vi "test_Tx Exec Unit (UDP).vi"() -> ()   [LabVIEW 2020]
uses:
  <instrlib>/AIM GmbH/_AIM 664/_controls/comm_config_vl_tx.ctl
  <instrlib>/AIM GmbH/_AIM 664/_controls/comm_udp_tx.ctl
  Shared/Encoding (Arinc664).ctl
  Import/_typedefs/board_setup.ctl
  <vilib>/NI VeriStand/Custom Device API/Custom Device Item Ref.ctl
  Engine/Implementation/Shared Resources/Shared Resources.lvclass
  C:/git/niveristand-aim-arinc664-custom-device/Source/Custom Device Support/Engine/Interfaces/Shared Resources/Shared Resources.lvclass
  Engine/Implementation/Tx UDP Execution Unit/Tx UDP Execution Unit.lvclass
  <vilib>/NI VeriStand/Custom Device API/Custom Device API.lvlib
  <instrlib>/AIM GmbH/_AIM 664/AIM664LV.lvlib
  Import/AIM ARINC 664 Import.lvlib
panel:
  in  "Tab Control":enum32{"Manual", "From File"}(tab)
  in  "tx_udp_vl":T3(array[cluster])=[{"VL Config"={"VlId"=60, "NumOfSubVl"=1, "rate ms [Bag]"=2, "domainID"=2, "sideID"=1, "locationID"=1, "interfaceID"=1, "NetSelect"=3, "Skew"=0, "MaxFrameLength"=559, "FrameBufferSize"=0}, "CommPort Config"=[{"PortType"=enum."FDX_UDP_SAMPLING", "partitionID"=1, "SubVlId"=1, "UdpSrcPort"=24, "UdpDstPort"=23, "SampleRateMs"=2.0, "UdpNumBufMessages"=0, "UdpMaxMessageSize"=512}, {"PortType"=enum."FDX_UDP_SAMPLING", "partitionID"=1, "SubVlId"=1, "UdpSrcPort"=34, "UdpDstPort"=33, "SampleRateMs"=2.0, "UdpNumBufMessages"=0, "UdpMaxMessageSize"=512}]}] {"VL Config"."NetSelect" items=["FDX_TX_FRAME_DLY_A"=0, "FDX_TX_FRAME_DLY_B"=1, "FDX_TX_FRAME_BOTH "=3, "FDX_TX_FRAME_ONLY_A"=4, "FDX_TX_FRAME_ONLY_B "=5]; "VL Config"."interfaceID" format="%.0b"}
  in  "tx_param":T5(array[cluster])=[{"Data"=[0, 0, 0, 0, 0, 0, 0, 0, 0, 0, 0, 0, 0, 0, 0, 0, 0, 0, 0, 0, 0, 0, 0, 0, 0, 0, 0, 0, 0, 0, 0, 0, 0, 0, 0, 0, 0, 0, 0, 0, 0, 0, 0, 0, 0, 0, 0, 0, 0, 0, 0, 0, 0, 0, 0, 0, 0, 0, 0, 0, 0, 0, 0, 0, 0, 0, 0, 0, 0, 0, 0, 0, 0, 0, 0, 0, 0, 0, 0, 0, 0, 0, 0, 0, 0, 0, 0, 0, 0, 0, 0, 0, 0, 0, 0, 0, 0, 0, 0, 0, 0, 0, 0, 0, 0, 0, 0, 0, 0, 0, 0, 0, 0, 0, 0, 0, 0, 0, 0, 0, 0, 0, 0, 0, 0, 0, 0, 0, 0, 0, 0, 0, 0, 0, 0, 0, 0, 0, 0, 0, 0, 0, 0, 0, 0, 0, 0, 0, 0, 0, 0, 0, 0, 0, 0, 0, 0, 0, 0, 0, 0, 0, 0, 0, 0, 0, 0, 0, 0, 0, 0, 0, 0, 0, 0, 0, 0, 0, 0, 0, 0, 0, 0, 0, 0, 0, 0, 0, 0, 0, 0, 0, 0, 0, 0, 0, 0, 0, 0, 0, 0, 0, 0, 0, 0, 0, 0, 0, 0, 0, 0, 0, 0, 0, 0, 0, 0, 0, 0, 0, 0, 0, 0, 0, 0, 0, 0, 0, 0, 0, 0, 0, 0, 0, 0, 0, 0, 0, 0, 0, 0, 0, 0, 0, 0, 0, 0, 0, 0, 0, 0, 0, 0, 0, 0, 0, 0, 0, 0, 0, 0, 0, 0, 0, 0, 0, 0, 0, 0, 0, 0, 0, 0, 0, 0, 0, 0, 0, 0, 0, 0, 0, 0, 0, 0, 0, 0, 0, 0, 0, 0, 0, 0, 0, 0, 0, 0, 0, 0, 0, 0, 0, 0, 0, 0, 0, 0, 0, 0, 0, 0, 0, 0, 0, 0, 0, 0, 0, 0, 0, 0, 0, 0, 0, 0, 0, 0, 0, 0, 0, 0, 0, 0, 0, 0, 0, 0, 0, 0, 0, 0, 0, 0, 0, 0, 0, 0, 0, 0, 0, 0, 0, 0, 0, 0, 0, 0, 0, 0, 0, 0, 0, 0, 0, 0, 0, 0, 0, 0, 0, 0, 0, 0, 0, 0, 0, 0, 0, 0, 0, 0, 0, 0, 0, 0, 0, 0, 0, 0, 0, 0, 0, 0, 0, 0, 0, 0, 0, 0, 0, 0, 0, 0, 0, 0, 0, 0, 0, 0, 0, 0, 0, 0, 0, 0, 0, 0, 0, 0, 0, 0, 0, 0, 0, 0, 0, 0, 0, 0, 0, 0, 0, 0, 0, 0, 0, 0, 0, 0, 0, 0, 0, 0, 0, 0, 0, 0, 0, 0, 0, 0, 0, 0, 0, 0, 0, 0, 0, 0, 0, 0, 0, 0, 0, 0, 0, 0, 0, 0, 0, 0, 0, 0, 0, 0, 0, 0, 0, 0, 0, 0, 0, 0, 0, 0, 0, 0, 0, 0, 0, 0, 0, 0, 0, 0, 0, 0, 0, 0, 0, 0, 0, 0, 0, 0, 0, 0, 0, 0, 0, 0, 0], "Parameters"=[{"start index"=0, "size"=64, "encoding"=6, "signed"=TRUE, "scale multiplier"=1.0, "scale offset"=0.0}, {"start index"=64, "size"=64, "encoding"=6, "signed"=TRUE, "scale multiplier"=1.0, "scale offset"=0.0}]}, {"Data"=[0, 0, 0, 0, 0, 0, 0, 0, 0, 0, 0, 0, 0, 0, 0, 0, 0, 0, 0, 0, 0, 0, 0, 0, 0, 0, 0, 0, 0, 0, 0, 0, 0, 0, 0, 0, 0, 0, 0, 0, 0, 0, 0, 0, 0, 0, 0, 0, 0, 0, 0, 0, 0, 0, 0, 0, 0, 0, 0, 0, 0, 0, 0, 0, 0, 0, 0, 0, 0, 0, 0, 0, 0, 0, 0, 0, 0, 0, 0, 0, 0, 0, 0, 0, 0, 0, 0, 0, 0, 0, 0, 0, 0, 0, 0, 0, 0, 0, 0, 0, 0, 0, 0, 0, 0, 0, 0, 0, 0, 0, 0, 0, 0, 0, 0, 0, 0, 0, 0, 0, 0, 0, 0, 0, 0, 0, 0, 0, 0, 0, 0, 0, 0, 0, 0, 0, 0, 0, 0, 0, 0, 0, 0, 0, 0, 0, 0, 0, 0, 0, 0, 0, 0, 0, 0, 0, 0, 0, 0, 0, 0, 0, 0, 0, 0, 0, 0, 0, 0, 0, 0, 0, 0, 0, 0, 0, 0, 0, 0, 0, 0, 0, 0, 0, 0, 0, 0, 0, 0, 0, 0, 0, 0, 0, 0, 0, 0, 0, 0, 0, 0, 0, 0, 0, 0, 0, 0, 0, 0, 0, 0, 0, 0, 0, 0, 0, 0, 0, 0, 0, 0, 0, 0, 0, 0, 0, 0, 0, 0, 0, 0, 0, 0, 0, 0, 0, 0, 0, 0, 0, 0, 0, 0, 0, 0, 0, 0, 0, 0, 0, 0, 0, 0, 0, 0, 0, 0, 0, 0, 0, 0, 0, 0, 0, 0, 0, 0, 0, 0, 0, 0, 0, 0, 0, 0, 0, 0, 0, 0, 0, 0, 0, 0, 0, 0, 0, 0, 0, 0, 0, 0, 0, 0, 0, 0, 0, 0, 0, 0, 0, 0, 0, 0, 0, 0, 0, 0, 0, 0, 0, 0, 0, 0, 0, 0, 0, 0, 0, 0, 0, 0, 0, 0, 0, 0, 0, 0, 0, 0, 0, 0, 0, 0, 0, 0, 0, 0, 0, 0, 0, 0, 0, 0, 0, 0, 0, 0, 0, 0, 0, 0, 0, 0, 0, 0, 0, 0, 0, 0, 0, 0, 0, 0, 0, 0, 0, 0, 0, 0, 0, 0, 0, 0, 0, 0, 0, 0, 0, 0, 0, 0, 0, 0, 0, 0, 0, 0, 0, 0, 0, 0, 0, 0, 0, 0, 0, 0, 0, 0, 0, 0, 0, 0, 0, 0, 0, 0, 0, 0, 0, 0, 0, 0, 0, 0, 0, 0, 0, 0, 0, 0, 0, 0, 0, 0, 0, 0, 0, 0, 0, 0, 0, 0, 0, 0, 0, 0, 0, 0, 0, 0, 0, 0, 0, 0, 0, 0, 0, 0, 0, 0, 0, 0, 0, 0, 0, 0, 0, 0, 0, 0, 0, 0, 0, 0, 0, 0, 0, 0, 0, 0, 0, 0, 0, 0, 0, 0, 0, 0, 0, 0, 0, 0, 0, 0, 0, 0, 0, 0, 0, 0, 0, 0, 0, 0, 0, 0, 0, 0, 0, 0, 0, 0, 0, 0, 0, 0, 0, 0, 0, 0, 0], "Parameters"=[{"start index"=0, "size"=64, "encoding"=6, "signed"=TRUE, "scale multiplier"=1.0, "scale offset"=0.0}, {"start index"=64, "size"=64, "encoding"=6, "signed"=TRUE, "scale multiplier"=1.0, "scale offset"=0.0}]}] {"Parameters"."encoding" items=["BNR", "BCD", "Discrete"]}
  in  "Tx_UDP_Frames file path":path=path "/home/admin/Port_0_Tx_UDP_Frames.bin"
  out "Frame parse error":errorcluster caption="error out"
  in  "Tx_UDP_VLs file path":path=path "/home/admin/Port_0_Tx_UDP_VLs.bin"
  in  "Update data every N calls":i32=1
  out "# of outs":i32=1
  in  "# of ins":i32=1
  out "exec time us":cluster{u32, u32}(graph)={659, 311}
  in  "Init Shared Resources":bool=TRUE
  in  "shared resources":T6 {"portConfig" items=["FDX_SINGLE", "FDX_REDUNDANT"]; "portSpeed" items=["FDX_100MBIT", "FDX_10MBIT", "FDX_AUTO_100MBIT", "FDX_AUTO_10MBIT", "FDX_AUTO_ERROR", "FDX_1000MBIT"]}
  in  "new element/subarray":dbl[](array[numeric])
  in  "port id":u32
  in  "board id":u32
  in  "loop rate mS":u32=10
  in  "stop":bool
  out "Values out":dbl[](array[numeric])=[1.0]
  out "error out":errorcluster
  # "Once running, switch to Manual tabl to see what has been uploaded from file"
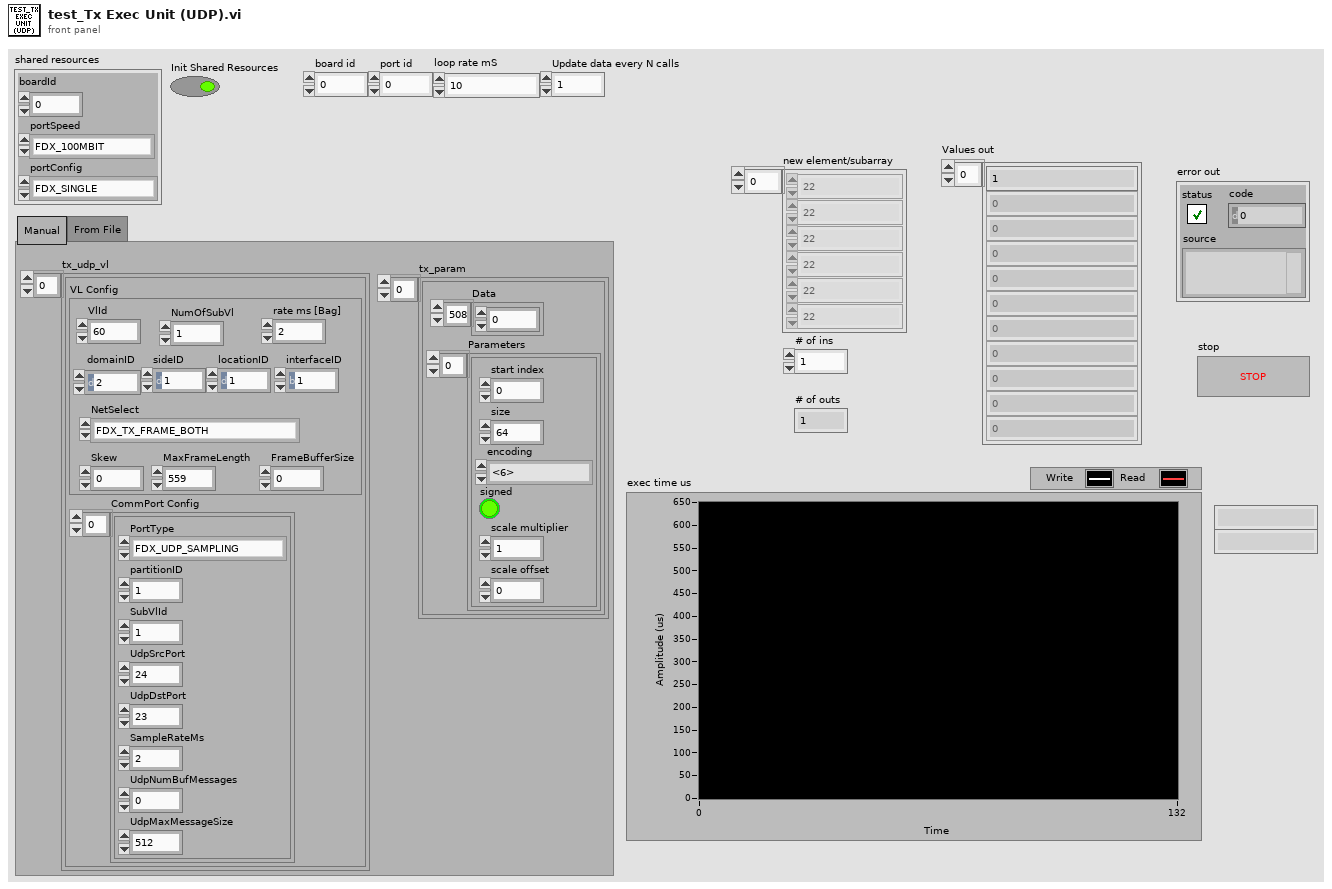
[diagram p1: front panel]
types:
  T1 = typedef "AIM664LV.lvlib/comm_config_vl_tx.ctl" = cluster{"VlId":u16, "NumOfSubVl":u16, "rate ms [Bag]":u32, "domainID":u8, "sideID":u8, "locationID":u8, "interfaceID":u8, "NetSelect":u32, "Skew":u32, "MaxFrameLength":u32, "FrameBufferSize":u32}
  T2 = typedef "AIM664LV.lvlib/comm_udp_tx.ctl" = cluster{"PortType":enum16{"FDX_UDP_SAMPLING", "FDX_UDP_QUEUING"}, "partitionID":u8, "SubVlId":u8, "UdpSrcPort":u16, "UdpDstPort":u16, "SampleRateMs":dbl, "UdpNumBufMessages":u32, "UdpMaxMessageSize":u32}
  T3 = cluster{"VL Config":T1, "CommPort Config":T2[]}[]
  T4 = typedef "Encoding (Arinc664).ctl" = u16
  T5 = cluster{"Data":u8[], "Parameters":cluster{"start index":i32, "size":i32, "encoding":T4, "signed":bool, "scale multiplier":dbl, "scale offset":dbl}[]}[]
  T6 = typedef "AIM ARINC 664 Import.lvlib/board_setup.ctl" = cluster{"boardId":u32, "portSpeed":u32, "portConfig":u32}
  T7 = typedef "Custom Device API.lvlib/Custom Device Item Ref.ctl" = u64
  T8 = cluster{"start index":i32, "size":i32, "encoding":T4, "signed":bool, "scale multiplier":dbl, "scale offset":dbl}[]
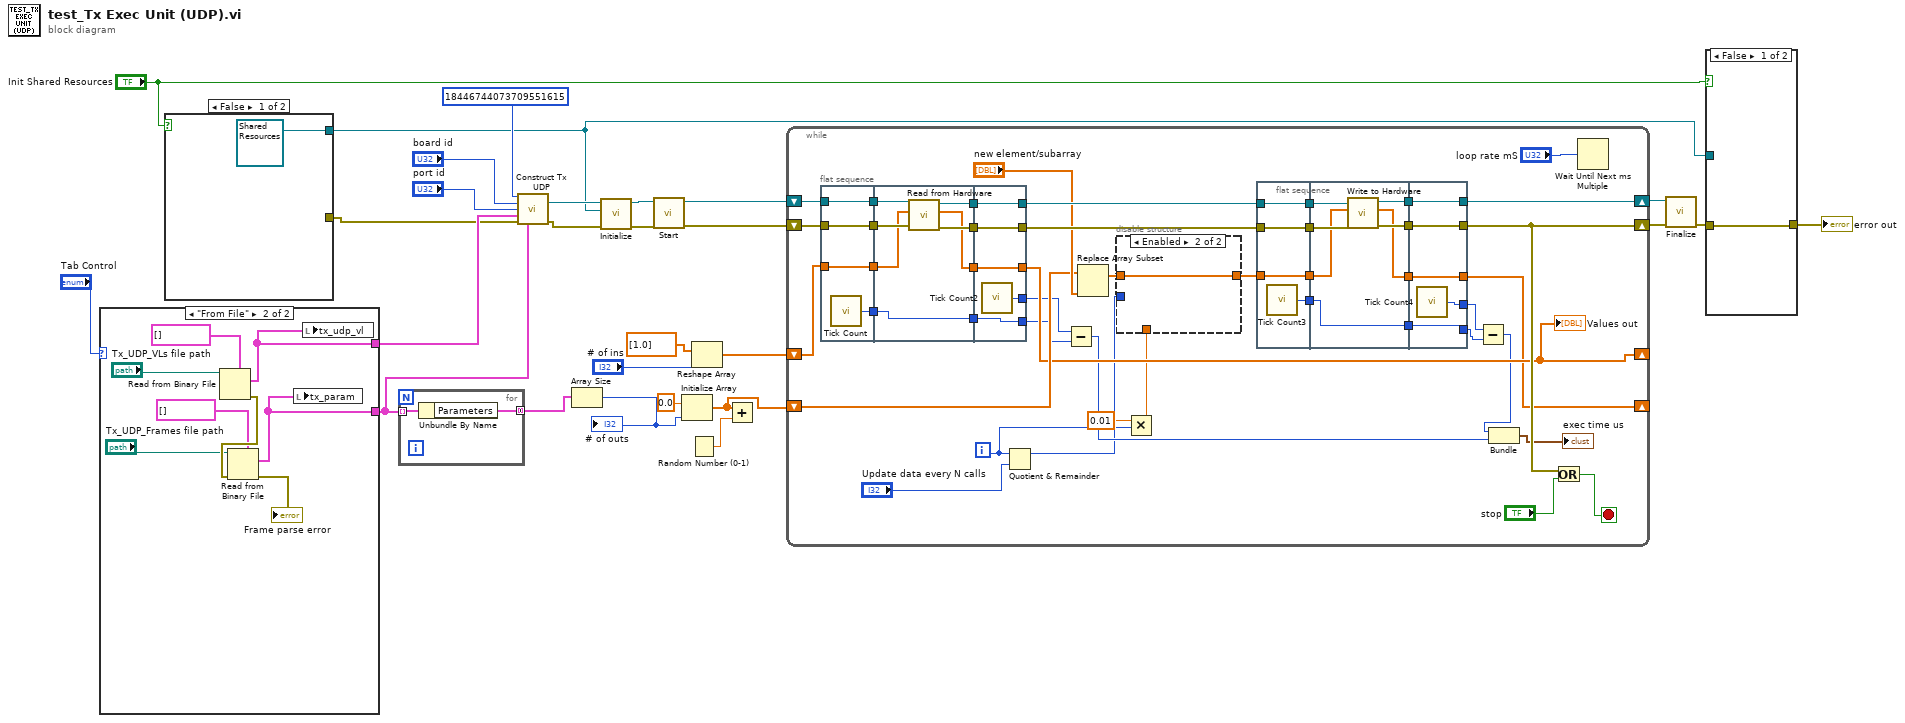
[diagram p0: block diagram]
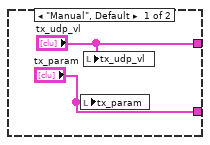
[diagram p2: hidden frame]
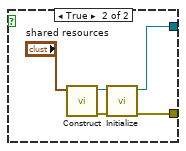
[diagram p3: hidden frame]
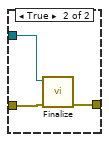
[diagram p4: hidden frame]
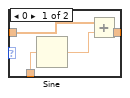
[diagram p6: hidden frame]
diagram:
  n1 = case shown="\"From File\"" "Tab Control" {
    tunnel: ["tx_udp_vl" w31] -> w18
    tunnel: ["tx_param" w30] -> w2
    frame "Manual", Default {
      n2 = local write "tx_param"("tx_param") -> ()
      n3 = local write "tx_udp_vl"("tx_udp_vl") -> ()
    }
    frame "From File" {
      n4 = Read from Binary File(5:T3 [] ("tx_udp_vl"), 11:"Tx_UDP_VLs file path") -> (0:w36:errorcluster, 2:w31:T3)  [unwired: 4 in, 2 out]
      n5 = Read from Binary File(5:T5 [] ("tx_param"), 8:w36, 11:"Tx_UDP_Frames file path") -> (0:→"Frame parse error":errorcluster, 2:w30:T5)  [unwired: 3 in, 2 out]
      n6 = local write "tx_param"(w30) -> ()
      n7 = local write "tx_udp_vl"(w31) -> ()
    }
  }
  n8 = case shown="False" "Init Shared Resources" {
    tunnel: [refnum<class "Shared Resources.lvclass"> refnum ("Shared Resources out") w41] -> w11
    tunnel: [_ w40] -> w15
    frame False {
    }
    frame True {
      n9 = call "Construct.vi"("board properties in"="shared resources") -> ("error out"=w42:errorcluster, "Shared Resources out"=w43:refnum<class "Shared Resources.lvclass">)  [unwired: 9 in]
      n10 = call-dynamic "Initialize.vi"("error in"=w42, "Shared Resources in"=w43) -> ("error out"=w40:errorcluster, "Shared Resources out"=w41:refnum<class "Shared Resources.lvclass">)  [unwired: 8 in]
    }
  }
  n11 = for {
    tunnel: [w45] -> w8 mode=concatenating
    tunnel: w2 -> [w44] mode=indexing
    n12 = Unbundle By Name(w44) -> ("Parameters"=w45:T8)
  }
  n13 = call "Construct Tx UDP.vi"("custom device ref in"=T7 18446744073709551615, "InstrumentHandle_board"="board id", "InstrumentHandle_port"="port id", "VL Configurations"=w18, "error in (no error)"=w15, "CommPort Payload"=w2) -> ("Execution Unit Out"=w21:refnum<class "Tx UDP Execution Unit.lvclass">, "error out"=w20:errorcluster)  [unwired: 7 in, 1 out]
  n14 = Array Size(array=w8) -> (size(s)=w7:i32)
  "# of outs" <- w7
  n15 = call-dynamic "Initialize.vi"("error in"=w20, "shared resources"=w11, "Tx UDP Execution Unit in"=w21) -> ("error out"=w27:errorcluster, "Tx UDP Execution Unit out"=w22:refnum<class "Tx UDP Execution Unit.lvclass">)  [unwired: 7 in]
  n16 = call-dynamic "Start.vi"("error in"=w27, "Tx UDP Execution Unit in"=w22) -> ("error out"=w24:errorcluster, "Tx UDP Execution Unit out"=w23:refnum<class "Tx UDP Execution Unit.lvclass">)  [unwired: 8 in]
  n17 = Initialize Array(0.0 ("Value"), w7) -> (w4:dbl[])
  n18 = Random Number (0-1)() -> (number: 0 to 1=w5:dbl)
  n19 = Reshape Array(dbl[] [1.0] ("Values in"), "# of ins") -> (w9:dbl[])
  n20 = Add(x=w4, y=w5) -> ()  [unwired: 1 out]
  n21 = while {
    shift-right: [w85] -> w25
    shift-left: w23 -> [w89]
    shift-right: [w83] -> w26
    shift-left: w24 -> [w88]
    shift-right: [w70] -> _
    shift-left: w9 -> [w73]
    shift-right: [w63] -> _
    shift-left: w4 -> [w74]
    i -> [w48]
    stop <- w81 stop-if-true
    n22 = flat-sequence {
      tunnel: w88 -> [w102]
      tunnel: w89 -> [w103]
      tunnel: [w103] -> w78
      tunnel: [w102] -> w77
      tunnel: w73 -> [w101]
      tunnel: [w101] -> w72
      tunnel: [w100] -> w59
      tunnel: w78 -> [w110]
      tunnel: w77 -> [w109]
      tunnel: [w108] -> w76
      tunnel: [w107] -> w75
      tunnel: w72 -> [w106]
      tunnel: [w105] -> w71
      tunnel: [w104] -> w60
      tunnel: w59 -> [w104]
      tunnel: [w114] -> w86
      tunnel: [w115] -> w87
      tunnel: w76 -> [w115]
      tunnel: w75 -> [w114]
      tunnel: [w113] -> w70
      tunnel: w71 -> [w113]
      tunnel: [w112] -> w62
      tunnel: [w111] -> w61
      tunnel: w60 -> [w111]
      frame #0 {
        n23 = call "Tick Count"() -> ("Tick Count(uSec)"=w100:u32)
      }
      frame #1 {
        n24 = call-dynamic "Read from Hardware.vi"("error in"=w109, "Values in"=w106, "Tx UDP Execution Unit in"=w110) -> ("error out"=w107:errorcluster, "Values out"=w105:dbl[], "Tx UDP Execution Unit out"=w108:refnum<class "Tx UDP Execution Unit.lvclass">)  [unwired: 6 in]
      }
      frame #2 {
        n25 = call "Tick Count2"() -> ("Tick Count(uSec)"=w112:u32)
      }
    }
    n26 = Quotient & Remainder(x=w48, y="Update data every N calls") -> (x-y*floor(x/y)=w49:i32)  [unwired: 1 out]
    n27 = Subtract(x=w62, y=w61) -> (x-y=w53:u32)
    n28 = Replace Array Subset(array=w74, new element="new element/subarray") -> (w80:dbl[])  [unwired: 1 in]
    n29 = Multiply(x=0.01, y=w48) -> (x*y=w47:dbl)
    n30 = disable-structure shown="Enabled" {
      disable-tunnel: w80 -> [w93 w99]
      disable-tunnel: [w92 w99] -> w51
      disable-tunnel: w49 -> [w91 _]
      disable-tunnel: w47 -> [w90 _]
      frame Disabled {
        n31 = case shown="1, Default" w91 {
          tunnel: w93 -> [w97 w98]
          tunnel: [w96 w98] -> w92
          tunnel: w90 -> [w94 _]
          frame 0 {
            n32 = Sine(x=w94) -> (sin(x)=w95:dbl)
            n33 = Add(x=w97, y=w95) -> (x+y=w96:dbl[])
          }
          frame 1, Default {
          }
        }
      }
      frame Enabled {
      }
    }
    n34 = flat-sequence {
      tunnel: w51 -> [w117]
      tunnel: w86 -> [w118]
      tunnel: w87 -> [w119]
      tunnel: [w119] -> w69
      tunnel: [w118] -> w68
      tunnel: [w117] -> w67
      tunnel: [w116] -> w57
      tunnel: w69 -> [w126]
      tunnel: w68 -> [w125]
      tunnel: w67 -> [w122]
      tunnel: [w124] -> w66
      tunnel: [w123] -> w65
      tunnel: [w121] -> w64
      tunnel: [w120] -> w58
      tunnel: w57 -> [w120]
      tunnel: [w130] -> w83
      tunnel: [w131] -> w85
      tunnel: w66 -> [w131]
      tunnel: w65 -> [w130]
      tunnel: [w129] -> w63
      tunnel: w64 -> [w129]
      tunnel: w58 -> [w127]
      tunnel: [w128] -> w56
      tunnel: [w127] -> w55
      frame #0 {
        n35 = call "Tick Count3"() -> ("Tick Count(uSec)"=w116:u32)
      }
      frame #1 {
        n36 = call-dynamic "Write to Hardware.vi"("error in"=w125, "Values in"=w122, "Tx UDP Execution Unit in"=w126) -> ("error out"=w123:errorcluster, "Values out"=w121:dbl[], "Tx UDP Execution Unit out"=w124:refnum<class "Tx UDP Execution Unit.lvclass">)  [unwired: 5 in, 1 out]
      }
      frame #2 {
        n37 = call "Tick Count4"() -> ("Tick Count(uSec)"=w128:u32)
      }
    }
    n38 = Subtract(x=w56, y=w55) -> (x-y=w54:u32)
    n39 = Bundle(w54, w53) -> (→"exec time us":cluster{u32, u32})  [unwired: 1 in]
    n40 = Or(x=w83, y="stop") -> (x .or. y?=w81:bool)
    n41 = Wait Until Next ms Multiple(millisecond multiple="loop rate mS") -> ()  [unwired: 1 out]
    "Values out" <- w70
  }
  n42 = call-dynamic "Finalize.vi"("error in"=w26, "Tx UDP Execution Unit in"=w25) -> ("error out"=w14:errorcluster)  [unwired: 8 in, 1 out]
  n43 = case shown="False" "Init Shared Resources" {
    tunnel: w14 -> [w132 w134]
    tunnel: [w132 w135] -> w13
    tunnel: w11 -> [_ w133]
    frame False {
    }
    frame True {
      n44 = call-dynamic "Finalize.vi"("error in"=w134, "Shared Resources in"=w133) -> ("error out"=w135:errorcluster)  [unwired: 8 in, 1 out]
    }
  }
  "error out" <- w13
